vi "Write to Disk.vi"(8 "error in (no error)":errorcluster, 10 "wfm dat in":waveform(cdb), 11 "tdms file":refnum<k34>) -> (0 "error out":errorcluster, 2 "wfm dat out":waveform(cdb), 3 "tdms file out":refnum<k34>, 5 "Bytes Analyzed per Second":dbl format="%#_5pB/sec")   [LabVIEW 2021]
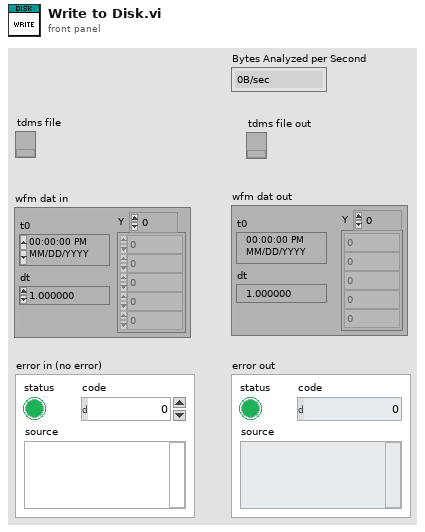
[diagram p1: front panel]
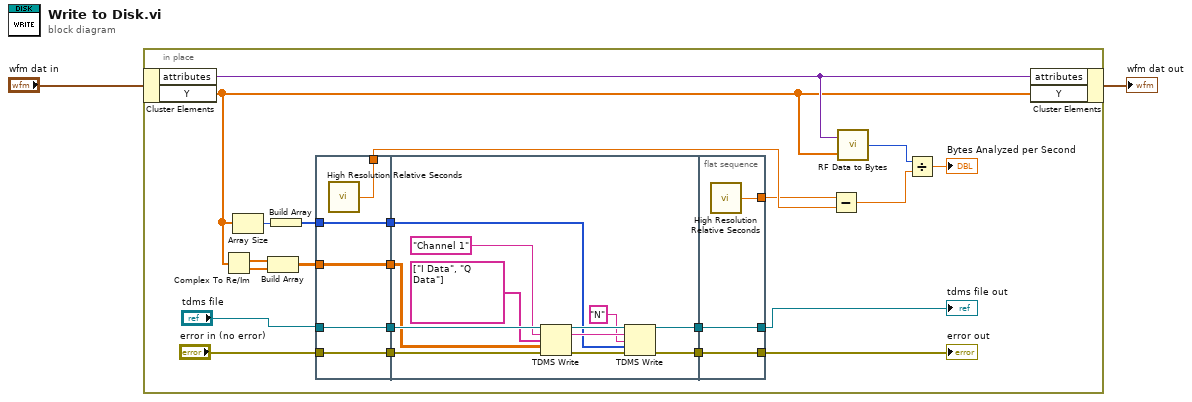
[diagram p0: block diagram]
diagram:
  n1 = in-place {
    n2 = in-place-cluster #1("wfm dat in") -> ("attributes"=w14:variant, "Y"=w7:cdb[])
    n3 = Complex To Re/Im(x + iy=w7) -> (x=w11:dbl[], y=w10:dbl[])
    n4 = Array Size(array=w7) -> (size(s)=w5:i32)
    n5 = Build Array(w11, w10) -> (w8:dbl[][])
    n6 = Build Array(w5) -> (w4:i32[])
    n7 = flat-sequence {
      tunnel: "tdms file" -> [w28]
      tunnel: "error in (no error)" -> [w29]
      tunnel: [w29] -> w24
      tunnel: [w28] -> w23
      tunnel: [w25] -> w18
      tunnel: [w27] -> w9
      tunnel: w8 -> [w27]
      tunnel: [w26] -> w6
      tunnel: w4 -> [w26]
      tunnel: [w35] -> w22
      tunnel: [w36] -> w21
      tunnel: w24 -> [w41]
      tunnel: w23 -> [w40]
      tunnel: w9 -> [w32]
      tunnel: w6 -> [w31]
      tunnel: [w43] -> w15
      tunnel: [w44] -> w16
      tunnel: w22 -> [w44]
      tunnel: w21 -> [w43]
      tunnel: [w42] -> w17
      frame #0 {
        n8 = call <vilib>:"High Resolution Relative Seconds.vi"() -> ("relative seconds"=w25:dbl)
      }
      frame #1 {
        n9 = TDMS Write(0:w40, 5:"Channel 1" ("group name in (Untitled)"), 7:string[] ["I Data", "Q Data"] ("channel name(s) in (Untitled)"), 9:w32, 11:w41) -> (4:w37:refnum<k34>, 6:w34:string, 15:w38:errorcluster)  [unwired: 1 in, 1 out]
        n10 = TDMS Write(0:w37, 5:w34, 7:"N" ("group name in (Untitled)"), 9:w31, 11:w38) -> (4:w36:refnum<k34>, 15:w35:errorcluster)  [unwired: 1 in, 2 out]
      }
      frame #2 {
        n11 = call <vilib>:"High Resolution Relative Seconds.vi"() -> ("relative seconds"=w42:dbl)
      }
    }
    n12 = Subtract(x=w17, y=w18) -> (x-y=w3:dbl)
    n13 = call "RF Data to Bytes.vi"("Y"=w7, "attributes"=w14) -> ("Bytes"=w19:i32)
    n14 = Divide(x=w19, y=w3) -> (x/y=→"Bytes Analyzed per Second":dbl)
    n15 = in-place-cluster #1("attributes"=w14, "Y"=w7) -> (→"wfm dat out":waveform(cdb))
    "error out" <- w16
    "tdms file out" <- w15
  }
